vi "TDM2TDMSData.vi"(0 "tdms file in":refnum<k34>, 5 "storage refnum in":refnum<k20>, 7 "group name":string="Random Numbers", 9 "channel name":string="Untitled", 11 "error in (no error)":errorcluster, 12 "chunk size":u32=10000000) -> (4 "tdms file out":refnum<k34>, 6 "storage refnum out":refnum<k20>, 8 "group name out":string="Random Numbers", 10 "channel name out":string="Untitled", 15 "error out":errorcluster)   [LabVIEW 2017]
doc: "Transfers data from the TDM storage to the TDMS file in chunks of a size specified in samples until all samples have been transferred."
uses:
  <vilib>/Utility/tdmsutil.llb/TDM2TDMSDatatypes.ctl
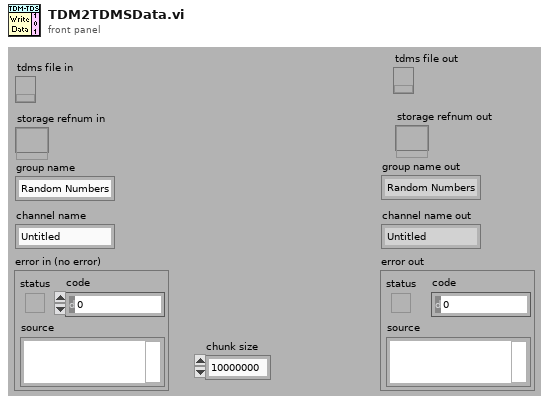
[diagram p1: front panel]
types:
  T1 = typedef "TDM2TDMSDatatypes.ctl" = enum16{"DT_UNKNOWN", "DT_STRING", "DT_SHORT", "DT_FLOAT", "DT_BOOLEAN", "DT_BYTE", "DT_LONG", "DT_DOUBLE", "DT_LONGLONG", "DT_ID", "DT_DATE", "DT_BYTESTR", "DT_BLOB", "DT_COMPLEX", "DT_DCOMPLEX", "DT_ENUM"}
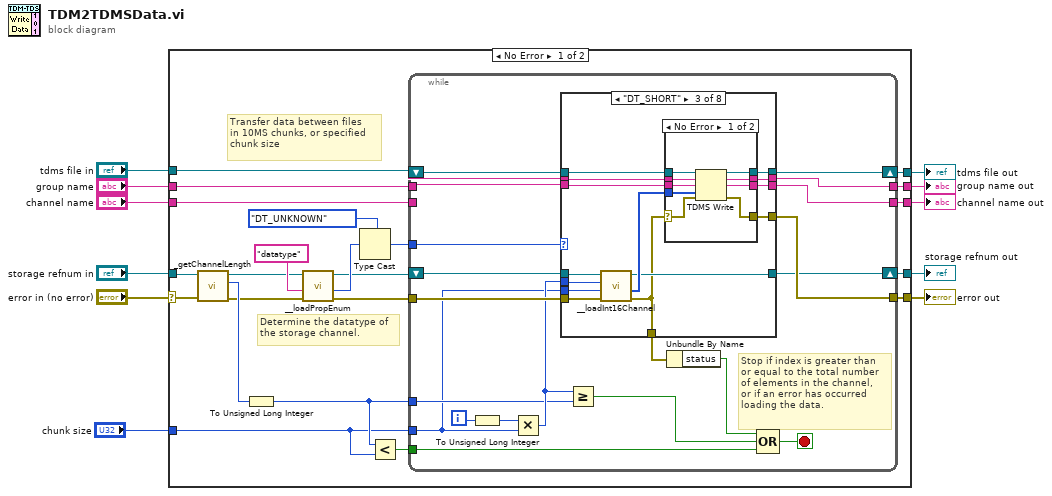
[diagram p0: block diagram]
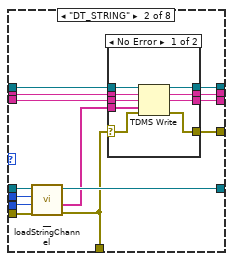
[diagram p3: hidden frame]
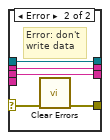
[diagram p4: hidden frame]
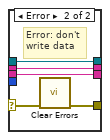
[diagram p5: hidden frame]
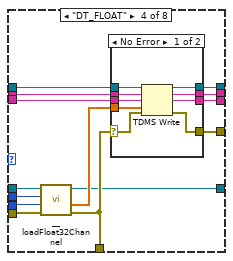
[diagram p6: hidden frame]
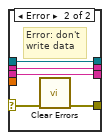
[diagram p7: hidden frame]
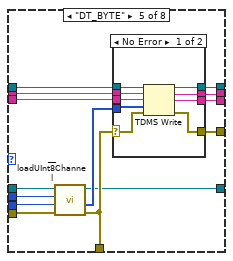
[diagram p8: hidden frame]
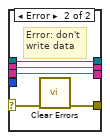
[diagram p9: hidden frame]
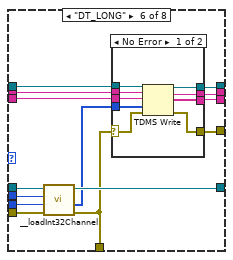
[diagram p10: hidden frame]
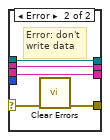
[diagram p11: hidden frame]
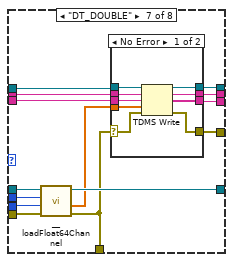
[diagram p12: hidden frame]
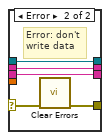
[diagram p13: hidden frame]
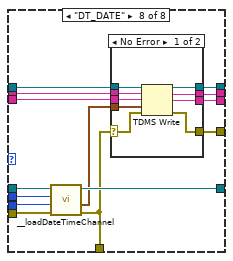
[diagram p14: hidden frame]
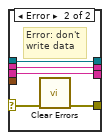
[diagram p15: hidden frame]
diagram:
  n1 = case shown="No Error" "error in (no error)" {
    selector: "error in (no error)" -> [w24 w258]
    tunnel: "channel name" -> [w32 w256]
    tunnel: "group name" -> [w31 w257]
    tunnel: [w30 w260] -> w7
    tunnel: "storage refnum in" -> [w25 w259]
    tunnel: "tdms file in" -> [w29 w260]
    tunnel: [w28 w259] -> w10
    tunnel: [w33 w258] -> w11
    tunnel: [w27 w257] -> w8
    tunnel: [w26 w256] -> w9
    tunnel: "chunk size" -> [w13 _]
    frame No Error {
      # "Determine the datatype of\nthe storage channel."
      # "Transfer data between files\nin 10MS chunks, or specified\nchunk size"
      n2 = call <vilib>:"_getChannelLength.vi"("error in (no error)"=w24, "channel refnum in"=w25) -> ("error out"=w18:errorcluster, "channel length"=w23:i32, "channel refnum out"=w19:refnum<k20>)  [unwired: 3 in]
      n3 = To Unsigned Long Integer(number=w23) -> (unsigned 32bit integer=w14:u32)
      n4 = call <vilib>:"__loadPropEnum.vi"("error in (no error)"=w18, "Property name"="datatype", "storage refnum"=w19) -> ("error out"=w16:errorcluster, "Value"=w20:u16, "dup storage refnum"=w17:refnum<k20>)  [unwired: 5 in, 1 out]
      n5 = Type Cast(type=TDM2TDMSDatatypes."DT_UNKNOWN" ("Data type"), x=w20) -> (*(type *) &x=w15:T1)
      n6 = Less?(x=w14, y=w13) -> (x < y?=w12:bool)
      n7 = while {
        tunnel: w31 -> [w53]
        tunnel: w32 -> [w52]
        shift-right: [w54] -> w30
        shift-left: w29 -> [w50]
        shift-right: [w39] -> w28
        shift-left: w17 -> [w42]
        tunnel: [w49] -> w33
        tunnel: [w48] -> w27
        tunnel: [w47] -> w26
        tunnel: w14 -> [w36]
        tunnel: w13 -> [w35]
        tunnel: w16 -> [w43]
        tunnel: w15 -> [w44]
        tunnel: w12 -> [w34]
        i -> [w46]
        stop <- w51 stop-if-true
        # "Stop if index is greater than\nor equal to the total number\nof elements in the channel,\nor if an error has occurred\nloading the data."
        n8 = To Unsigned Long Integer(number=w46) -> (unsigned 32bit integer=w45:u32)
        n9 = Multiply(x=w45, y=w35) -> (x*y=w40:u32)
        n10 = case shown="\"DT_SHORT\"" w44 {
          tunnel: [w59 w73 w100 w124 w157 w182 w208 w241] -> w54
          tunnel: w53 -> [w58 w72 w99 w123 w155 w175 w201 w231]
          tunnel: w52 -> [w55 w71 w98 w122 w154 w174 w200 w230]
          tunnel: w50 -> [w59 w70 w101 w125 w156 w176 w202 w232]
          tunnel: [w57 w69 w91 w119 w147 w179 w205 w228] -> w49
          tunnel: [w58 w68 w89 w117 w145 w181 w207 w240] -> w48
          tunnel: [w55 w60 w88 w116 w144 w180 w206 w229] -> w47
          tunnel: w43 -> [w57 w66 w96 w128 w152 w184 w212 w238]
          tunnel: w42 -> [w56 w67 w97 w129 w153 w185 w213 w239]
          tunnel: w40 -> [_ w65 w95 w127 w151 w173 w211 w237]
          tunnel: w35 -> [_ w64 w94 w126 w150 w172 w210 w236]
          tunnel: [w56 w63 w92 w118 w146 w183 w209 w235] -> w39
          tunnel: [w57 w61 w90 w120 w148 w177 w204 w234] -> w38
          frame "DT_UNKNOWN", Default {
          }
          frame "DT_STRING" {
            n11 = call <vilib>:"__loadStringChannel.vi"("error in (no error)"=w66, "Count"=w64, "Index"=w65, "Data object in"=w67) -> ("error out"=w61:errorcluster, "Values"=w62:string[], "Data object out"=w63:refnum<k20>)  [unwired: 1 out]
            n12 = case shown="No Error" w61 {
              tunnel: [w82 w87] -> w73
              tunnel: w72 -> [w81 w86]
              tunnel: w71 -> [w75 w83]
              tunnel: w70 -> [w80 w87]
              tunnel: [w79 w84] -> w69
              selector: w61 -> [w78 w85]
              tunnel: [w77 w86] -> w68
              tunnel: [w76 w83] -> w60
              tunnel: w62 -> [w74 _]
              frame No Error {
                n13 = TDMS Write(0:w80, 5:w81, 7:w75, 9:w74, 11:w78) -> (4:w82:refnum<k34>, 6:w77:string, 8:w76:string, 15:w79:errorcluster)  [unwired: 1 in]
              }
              frame Error {
                # "Error: don't\nwrite data"
                n14 = call <vilib>:"Clear Errors.vi"("error in (no error)"=w85) -> ("error out"=w84:errorcluster)  [unwired: 5 in, 1 out]
              }
            }
          }
          frame "DT_SHORT" {
            n15 = call <vilib>:"__loadInt16Channel.vi"("error in (no error)"=w96, "Count"=w94, "Index"=w95, "Data object in"=w97) -> ("error out"=w90:errorcluster, "Values"=w93:i16[], "Data object out"=w92:refnum<k20>)  [unwired: 1 out]
            n16 = case shown="No Error" w90 {
              tunnel: [w110 w115] -> w100
              tunnel: w99 -> [w109 w114]
              tunnel: w98 -> [w103 w111]
              tunnel: w101 -> [w108 w115]
              tunnel: [w107 w112] -> w91
              selector: w90 -> [w106 w113]
              tunnel: [w105 w114] -> w89
              tunnel: [w104 w111] -> w88
              tunnel: w93 -> [w102 _]
              frame No Error {
                n17 = TDMS Write(0:w108, 5:w109, 7:w103, 9:w102, 11:w106) -> (4:w110:refnum<k34>, 6:w105:string, 8:w104:string, 15:w107:errorcluster)  [unwired: 1 in]
              }
              frame Error {
                # "Error: don't\nwrite data"
                n18 = call <vilib>:"Clear Errors.vi"("error in (no error)"=w113) -> ("error out"=w112:errorcluster)  [unwired: 5 in, 1 out]
              }
            }
          }
          frame "DT_FLOAT" {
            n19 = call <vilib>:"__loadFloat32Channel.vi"("error in (no error)"=w128, "Count"=w126, "Index"=w127, "Data object in"=w129) -> ("error out"=w120:errorcluster, "Values"=w121:sgl[], "Data object out"=w118:refnum<k20>)  [unwired: 1 in]
            n20 = case shown="No Error" w120 {
              tunnel: [w138 w143] -> w124
              tunnel: w123 -> [w137 w142]
              tunnel: w122 -> [w131 w139]
              tunnel: w125 -> [w136 w143]
              tunnel: [w135 w140] -> w119
              selector: w120 -> [w134 w141]
              tunnel: [w133 w142] -> w117
              tunnel: [w132 w139] -> w116
              tunnel: w121 -> [w130 _]
              frame No Error {
                n21 = TDMS Write(0:w136, 5:w137, 7:w131, 9:w130, 11:w134) -> (4:w138:refnum<k34>, 6:w133:string, 8:w132:string, 15:w135:errorcluster)  [unwired: 1 in]
              }
              frame Error {
                # "Error: don't\nwrite data"
                n22 = call <vilib>:"Clear Errors.vi"("error in (no error)"=w141) -> ("error out"=w140:errorcluster)  [unwired: 5 in, 1 out]
              }
            }
          }
          frame "DT_BYTE" {
            n23 = call <vilib>:"__loadUInt8Channel.vi"("error in (no error)"=w152, "Count"=w150, "Index"=w151, "Data object in"=w153) -> ("error out"=w148:errorcluster, "Values"=w149:u8[], "Data object out"=w146:refnum<k20>)  [unwired: 1 out]
            n24 = case shown="No Error" w148 {
              tunnel: [w166 w169] -> w157
              tunnel: [w165 w170] -> w147
              selector: w148 -> [w164 w171]
              tunnel: [w163 w168] -> w145
              tunnel: [w162 w167] -> w144
              tunnel: w156 -> [w161 w169]
              tunnel: w155 -> [w160 w168]
              tunnel: w154 -> [w159 w167]
              tunnel: w149 -> [w158 _]
              frame No Error {
                n25 = TDMS Write(0:w161, 5:w160, 7:w159, 9:w158, 11:w164) -> (4:w166:refnum<k34>, 6:w163:string, 8:w162:string, 15:w165:errorcluster)  [unwired: 1 in]
              }
              frame Error {
                # "Error: don't\nwrite data"
                n26 = call <vilib>:"Clear Errors.vi"("error in (no error)"=w171) -> ("error out"=w170:errorcluster)  [unwired: 5 in, 1 out]
              }
            }
          }
          frame "DT_LONG" {
            n27 = call <vilib>:"__loadInt32Channel.vi"("error in (no error)"=w184, "Count"=w172, "Index"=w173, "Data object in"=w185) -> ("error out"=w177:errorcluster, "Values"=w178:i32[], "Data object out"=w183:refnum<k20>)  [unwired: 1 out]
            n28 = case shown="No Error" w177 {
              tunnel: [w194 w197] -> w182
              tunnel: [w193 w198] -> w179
              selector: w177 -> [w192 w199]
              tunnel: [w191 w196] -> w181
              tunnel: [w190 w195] -> w180
              tunnel: w178 -> [w189 _]
              tunnel: w176 -> [w188 w197]
              tunnel: w175 -> [w187 w196]
              tunnel: w174 -> [w186 w195]
              frame No Error {
                n29 = TDMS Write(0:w188, 5:w187, 7:w186, 9:w189, 11:w192) -> (4:w194:refnum<k34>, 6:w191:string, 8:w190:string, 15:w193:errorcluster)  [unwired: 1 in]
              }
              frame Error {
                # "Error: don't\nwrite data"
                n30 = call <vilib>:"Clear Errors.vi"("error in (no error)"=w199) -> ("error out"=w198:errorcluster)  [unwired: 5 in, 1 out]
              }
            }
          }
          frame "DT_DOUBLE" {
            n31 = call <vilib>:"__loadFloat64Channel.vi"("error in (no error)"=w212, "Count"=w210, "Index"=w211, "Data object in"=w213) -> ("error out"=w204:errorcluster, "Values"=w203:dbl[], "Data object out"=w209:refnum<k20>)  [unwired: 1 out]
            n32 = case shown="No Error" w204 {
              tunnel: [w222 w225] -> w208
              tunnel: [w221 w226] -> w205
              selector: w204 -> [w220 w227]
              tunnel: [w219 w224] -> w207
              tunnel: [w218 w223] -> w206
              tunnel: w203 -> [w217 _]
              tunnel: w202 -> [w216 w225]
              tunnel: w201 -> [w215 w224]
              tunnel: w200 -> [w214 w223]
              frame No Error {
                n33 = TDMS Write(0:w216, 5:w215, 7:w214, 9:w217, 11:w220) -> (4:w222:refnum<k34>, 6:w219:string, 8:w218:string, 15:w221:errorcluster)  [unwired: 1 in]
              }
              frame Error {
                # "Error: don't\nwrite data"
                n34 = call <vilib>:"Clear Errors.vi"("error in (no error)"=w227) -> ("error out"=w226:errorcluster)  [unwired: 5 in, 1 out]
              }
            }
          }
          frame "DT_DATE" {
            n35 = call <vilib>:"__loadDateTimeChannel.vi"("error in (no error)"=w238, "Count"=w236, "Index"=w237, "Data object in"=w239) -> ("error out"=w234:errorcluster, "Values"=w233:timestamp[], "Data object out"=w235:refnum<k20>)  [unwired: 1 out]
            n36 = case shown="No Error" w234 {
              tunnel: [w250 w253] -> w241
              tunnel: [w249 w254] -> w228
              selector: w234 -> [w248 w255]
              tunnel: [w247 w252] -> w240
              tunnel: [w246 w251] -> w229
              tunnel: w233 -> [w245 _]
              tunnel: w232 -> [w244 w253]
              tunnel: w231 -> [w243 w252]
              tunnel: w230 -> [w242 w251]
              frame No Error {
                n37 = TDMS Write(0:w244, 5:w243, 7:w242, 9:w245, 11:w248) -> (4:w250:refnum<k34>, 6:w247:string, 8:w246:string, 15:w249:errorcluster)  [unwired: 1 in]
              }
              frame Error {
                # "Error: don't\nwrite data"
                n38 = call <vilib>:"Clear Errors.vi"("error in (no error)"=w255) -> ("error out"=w254:errorcluster)  [unwired: 5 in, 1 out]
              }
            }
          }
        }
        n39 = Greater Or Equal?(x=w40, y=w36) -> (x >= y?=w37:bool)
        n40 = Unbundle By Name(w38) -> ("status"=w41:bool)
        n41 = Compound Arithmetic op=OR(w41, w37, w34) -> (w51:bool)
      }
    }
    frame Error {
    }
  }
  "tdms file out" <- w7
  "storage refnum out" <- w10
  "error out" <- w11
  "group name out" <- w8
  "channel name out" <- w9
